vi "ConstantToArray_CDB.vi"(11 "Constant":cdb) -> (3 "ConstantArray":dbl[](array[numeric]))   [LabVIEW 2020, in "OpenLvVision_OpenCv.lvlib"]
uses:
  OpenLvVision_OpenCv.lvlib
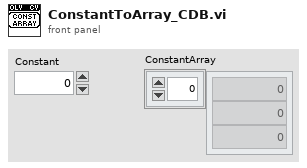
[diagram p1: front panel]
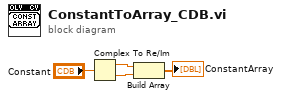
[diagram p0: block diagram]
diagram:
  n1 = Complex To Re/Im(x + iy="Constant") -> (x=w1:dbl, y=w2:dbl)
  n2 = Build Array(w1, w2) -> (→"ConstantArray":dbl[])
